vi "go to angle.vi"(6 "Pause Time [ms]":i32=50, 8 "error in (no error)":errorcluster, 9 "Velocity [rpm]":i32=5, 10 "Angle":dbl, 11 "Stepper in":refnum<class "Stepper.lvclass">) -> (0 "error out":errorcluster, 3 "Stepper out":refnum<class "Stepper.lvclass">)   [LabVIEW 2025, in "Motor.lvlib" / "Stepper.lvclass"]
uses:
  Stepper.lvclass
  Path Mode.ctl
  Stepper.lvclass/Stepper.ctl
  Motor.lvlib
panel:
  out "Running?":bool
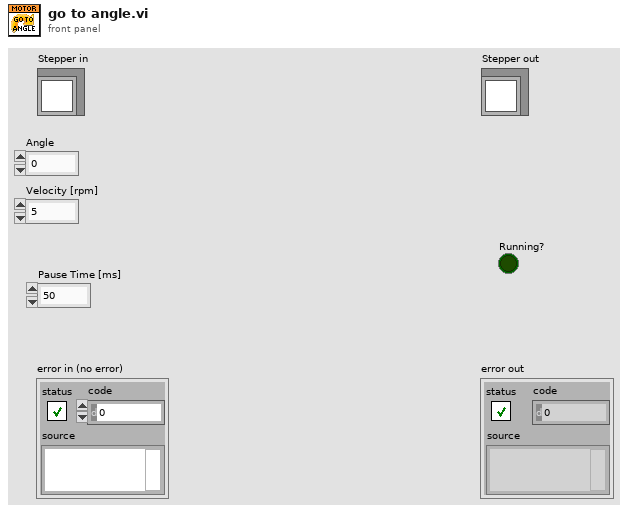
[diagram p1: front panel]
types:
  T1 = typedef "Motor.lvlib/Path Mode.ctl" = enum16{"Position Mode", "Velocity Mode", "Homing Mode"}
  T2 = cluster{"Path Number":i32, "Path Mode":T1, "Relative?":enum16{"Relative", "Absolute"}, "Angle":dbl, "Velocity [rpm]":i32, "Acceleration [ms/krpm]":i32, "Deceleration [ms/krpm]":i32, "Pause Time [ms]":i32}
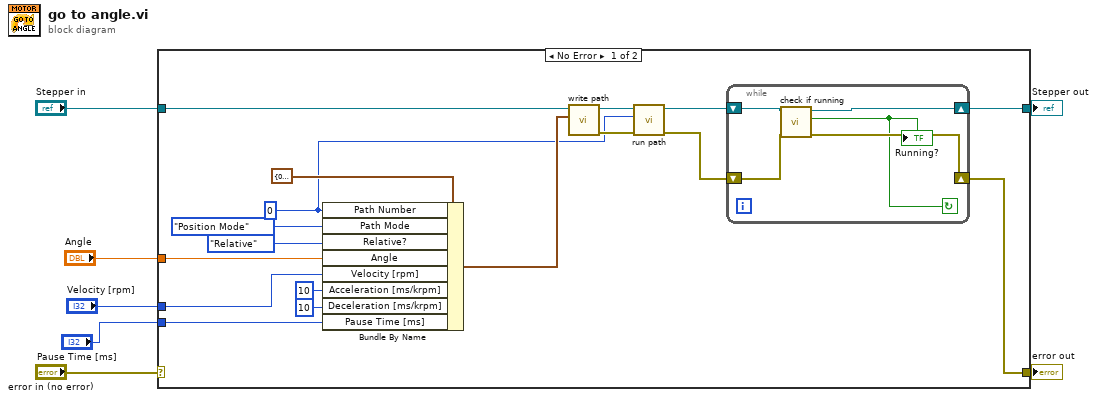
[diagram p0: block diagram]
diagram:
  n1 = case shown="No Error" "error in (no error)" {
    selector: "error in (no error)" -> [_ w31]
    tunnel: [w8 w31] -> w6
    tunnel: [w11 w30] -> w4
    tunnel: "Stepper in" -> [w13 w30]
    tunnel: "Angle" -> [w20 _]
    tunnel: "Velocity [rpm]" -> [w19 _]
    tunnel: "Pause Time [ms]" -> [w16 _]
    frame No Error {
      w12 = 0 ("Path Number")
      n2 = Bundle By Name(cluster=T2 {"Path Number"=0, "Path Mode"=enum."Position Mode", "Relative?"=enum."Relative", "Angle"=0.0, "Velocity [rpm]"=0, "Acceleration [ms/krpm]"=0, "Deceleration [ms/krpm]"=0, "Pause Time [ms]"=0} ("Path Cluster"), "Path Number"=w12, "Path Mode"=Path_Mode."Position Mode", "Relative?"=enum16{"Relative", "Absolute"}."Relative", "Angle"=w20, "Velocity [rpm]"=w19, "Acceleration [ms/krpm]"=10, "Deceleration [ms/krpm]"=10, "Pause Time [ms]"=w16) -> (w15:T2)
      n3 = call-dynamic "write path.vi"("Path Cluster"=w15, "Stepper in"=w13) -> ("error out"=w14:errorcluster, "Stepper out"=w24:refnum<class "Stepper.lvclass">)  [unwired: 8 in]
      n4 = call-dynamic "run path.vi"("error in (no error)"=w14, "Path Number"=w12, "Stepper in"=w24) -> ("error out"=w9:errorcluster, "Stepper out"=w10:refnum<class "Stepper.lvclass">)  [unwired: 7 in]
      n5 = while {
        shift-right: [w29] -> w11
        shift-left: w10 -> [w28]
        shift-right: [w26] -> w8
        shift-left: w9 -> [w27]
        stop <- w25 continue-if-true
        n6 = call-dynamic "check if running.vi"("error in (no error)"=w27, "Stepper in"=w28) -> ("error out"=w26:errorcluster, "Running?"=w25:bool, "Stepper out"=w29:refnum<class "Stepper.lvclass">)  [unwired: 7 in]
        "Running?" <- w25
      }
    }
    frame Error {
    }
  }
  "error out" <- w6
  "Stepper out" <- w4
